vi "Validate Channel Alias Name.vi"(11 "Channel Alias":string) -> (2 "Invalid Info":string, 3 "Valid?":bool)   [LabVIEW 2021]
uses:
  <vilib>/myRIO/Common/Express VI Framework/vis/Express VI Framework Strings Global.vi
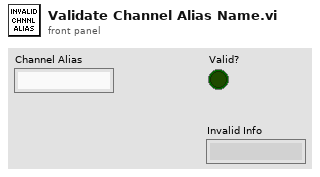
[diagram p1: front panel]
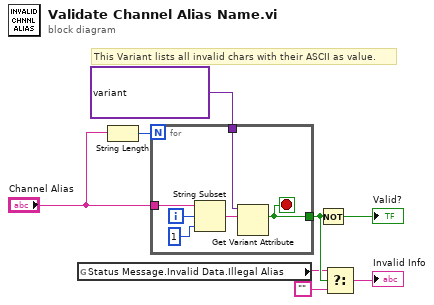
[diagram p0: block diagram]
diagram:
  # "This Variant lists all invalid chars with their ASCII as value."
  n1 = global read "Express VI Framework Strings Global.vi" "Status Message.Invalid Data.Illegal Alias"() -> (w3:string)
  n2 = String Length(string="Channel Alias") -> (length=w8:i32)
  n3 = for {
    N: w8 -> [_]
    tunnel: "Channel Alias" -> [w14]
    tunnel: [w10] -> w4
    tunnel: variant("\u0000"=variant(i32 0), "\u0001"=variant(i32 1), "\u0002"=variant(i32 2), "\u0003"=variant(i32 3), "\u0004"=variant(i32 4), "\u0005"=variant(i32 5), "\u0006"=variant(i32 6), "\u0007"=variant(i32 7), "\b"=variant(i32 8), "\u000b"=variant(i32 11), "\f"=variant(i32 12), "\u000e"=variant(i32 14), "\u000f"=variant(i32 15), "\u0010"=variant(i32 16), "\u0011"=variant(i32 17), "\u0012"=variant(i32 18), "\u0013"=variant(i32 19), "\u0014"=variant(i32 20), "\u0015"=variant(i32 21), "\u0016"=variant(i32 22), "\u0017"=variant(i32 23), "\u0018"=variant(i32 24), "\u0019"=variant(i32 25), "\u001a"=variant(i32 26), "\u001b"=variant(i32 27), "\u001c"=variant(i32 28), "\u001d"=variant(i32 29), "\u001e"=variant(i32 30), "\u001f"=variant(i32 31), "\""=variant(i32 34), "&"=variant(i32 38), "<"=variant(i32 60), "€"=variant(i32 128), ""=variant(i32 129), "‚"=variant(i32 130), "ƒ"=variant(i32 131), "„"=variant(i32 132), "…"=variant(i32 133), "†"=variant(i32 134), "‡"=variant(i32 135), "ˆ"=variant(i32 136), "‰"=variant(i32 137), "Š"=variant(i32 138), "‹"=variant(i32 139), "Œ"=variant(i32 140), ""=variant(i32 141), "Ž"=variant(i32 142), ""=variant(i32 143), ""=variant(i32 144), "‘"=variant(i32 145), "’"=variant(i32 146), "“"=variant(i32 147), "”"=variant(i32 148), "•"=variant(i32 149), "–"=variant(i32 150), "—"=variant(i32 151), "˜"=variant(i32 152), "™"=variant(i32 153), "š"=variant(i32 154), "›"=variant(i32 155), "œ"=variant(i32 156), ""=variant(i32 157), "ž"=variant(i32 158), "Ÿ"=variant(i32 159), " "=variant(i32 160), "¡"=variant(i32 161), "¢"=variant(i32 162), "£"=variant(i32 163), "¤"=variant(i32 164), "¥"=variant(i32 165), "¦"=variant(i32 166), "§"=variant(i32 167), "¨"=variant(i32 168), "©"=variant(i32 169), "ª"=variant(i32 170), "«"=variant(i32 171), "¬"=variant(i32 172), "­"=variant(i32 173), "®"=variant(i32 174), "¯"=variant(i32 175), "°"=variant(i32 176), "±"=variant(i32 177), "²"=variant(i32 178), "³"=variant(i32 179), "´"=variant(i32 180), "µ"=variant(i32 181), "¶"=variant(i32 182), "·"=variant(i32 183), "¸"=variant(i32 184), "¹"=variant(i32 185), "º"=variant(i32 186), "»"=variant(i32 187), "¼"=variant(i32 188), "½"=variant(i32 189), "¾"=variant(i32 190), "¿"=variant(i32 191), "À"=variant(i32 192), "Á"=variant(i32 193), "Â"=variant(i32 194), "Ã"=variant(i32 195), "Ä"=variant(i32 196), "Å"=variant(i32 197), "Æ"=variant(i32 198), "Ç"=variant(i32 199), "È"=variant(i32 200), "É"=variant(i32 201), "Ê"=variant(i32 202), "Ë"=variant(i32 203), "Ì"=variant(i32 204), "Í"=variant(i32 205), "Î"=variant(i32 206), "Ï"=variant(i32 207), "Ð"=variant(i32 208), "Ñ"=variant(i32 209), "Ò"=variant(i32 210), "Ó"=variant(i32 211), "Ô"=variant(i32 212), "Õ"=variant(i32 213), "Ö"=variant(i32 214), "×"=variant(i32 215), "Ø"=variant(i32 216), "Ù"=variant(i32 217), "Ú"=variant(i32 218), "Û"=variant(i32 219), "Ü"=variant(i32 220), "Ý"=variant(i32 221), "Þ"=variant(i32 222), "ß"=variant(i32 223), "à"=variant(i32 224), "á"=variant(i32 225), "â"=variant(i32 226), "ã"=variant(i32 227), "ä"=variant(i32 228), "å"=variant(i32 229), "æ"=variant(i32 230), "ç"=variant(i32 231), "è"=variant(i32 232), "é"=variant(i32 233), "ê"=variant(i32 234), "ë"=variant(i32 235), "ì"=variant(i32 236), "í"=variant(i32 237), "î"=variant(i32 238), "ï"=variant(i32 239), "ð"=variant(i32 240), "ñ"=variant(i32 241), "ò"=variant(i32 242), "ó"=variant(i32 243), "ô"=variant(i32 244), "õ"=variant(i32 245), "ö"=variant(i32 246), "÷"=variant(i32 247), "ø"=variant(i32 248), "ù"=variant(i32 249), "ú"=variant(i32 250), "û"=variant(i32 251), "ü"=variant(i32 252), "ý"=variant(i32 253), "þ"=variant(i32 254), "ÿ"=variant(i32 255)) ("Variant") -> [w9]
    i -> [w13]
    stop <- w10 stop-if-true
    n4 = String Subset(string=w14, offset (0)=w13, length (rest)=1 ("length (rest)")) -> (substring=w11:string)
    n5 = Get Variant Attribute(Variant=w9, name=w11) -> (found=w10:bool)  [unwired: 2 in, 3 out]
  }
  n6 = Not(x=w4) -> (.not. x?=→"Valid?":bool)
  n7 = Select(t=w3, s=w4, f="") -> (s? t:f=→"Invalid Info":string)
